vi "Pulse.vi"(8 "error in (no error)":errorcluster, 9 "Sender":string, 10 "Pulse In":enum16{"Low", "High"}(ring), 11 "Module In":refnum<class "Module.lvclass">) -> (0 "error out":errorcluster, 1 "Receivers":string[](array[string]), 2 "Pulse Out":enum16{"Low", "High"}(ring), 3 "Module Out":refnum<class "Module.lvclass">)   [LabVIEW 2021, in "Module.lvclass"]
uses:
  Module.lvclass
  Module.lvclass/Module.ctl
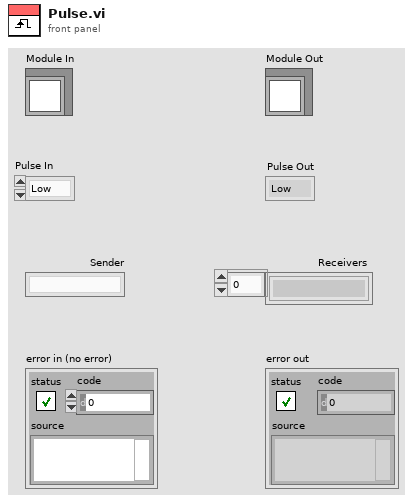
[diagram p1: front panel]
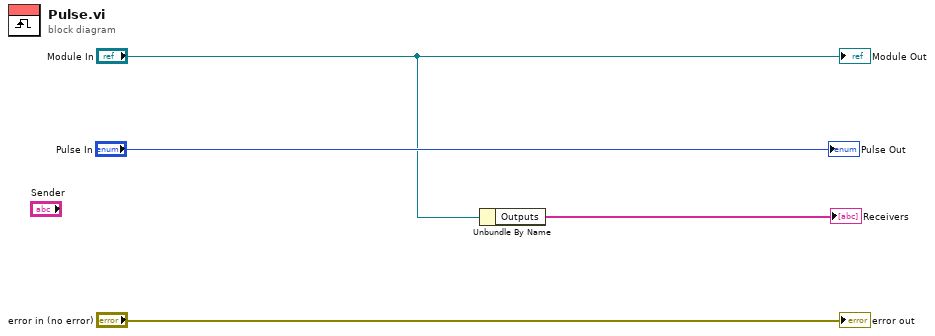
[diagram p0: block diagram]
diagram:
  n1 = Unbundle By Name("Module In") -> ("Outputs"=→"Receivers":string[])
  "error out" <- "error in (no error)"
  "Module Out" <- "Module In"
  "Pulse Out" <- "Pulse In"
